vi "get parameters.vi"(8 "error in (no error)":errorcluster, 11 "Request in":variant) -> (0 "error out":errorcluster, 1 "found?":bool, 2 "params":variant, 3 "Request out":variant)   [LabVIEW 2017, in "JSONRPC Server.lvclass"]
uses:
  JSONRPC Server.lvclass
  <vilib>/National Instruments/Variant Data Manipulation/Variant Data Manipulation.lvlib
  <vilib>/Utility/Data Type/NI_Data Type.lvlib
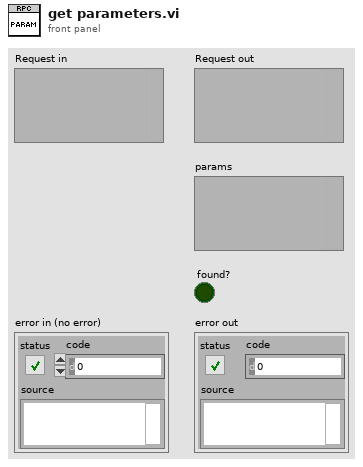
[diagram p1: front panel]
types:
  T1 = typedef "NI_Data Type.lvlib/Data Type.ctl" = enum8{"Invalid Type", "Void", "I8", "I16", "I32", "I64", "U8", "U16", "U32", "U64", "Single Float", "Double Float", "Extended Float", "Single Complex", "Double Complex", "Extended Complex", "Enum U8", "Enum U16", "Enum U32", "Enum U64", "Single Float With Unit", "Double Float With Unit", "Extended Float With Unit", "Single Complex with Unit", "Double Complex with Unit", "Extended Complex with Unit", "Boolean", "String", "Path", "Picture", "Tag", "Array", "Cluster", "Variant", "LV Variant", "Waveform", "Timestamp", "Digital Waveform", "Digital Data", "ExpressData", "Refnum", "External Data", "VI", "Poly VI", "LabVIEW Class Instance", "Fixed Point"}
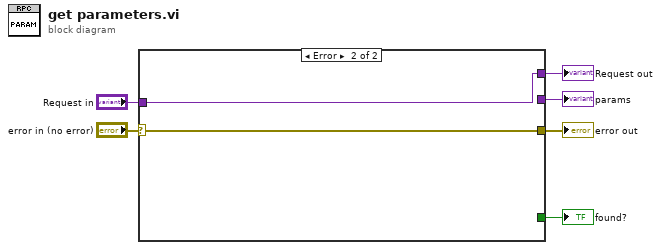
[diagram p0: block diagram]
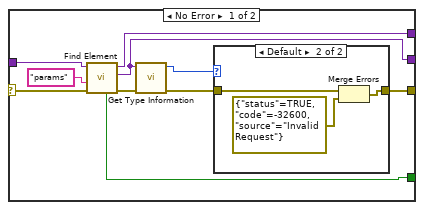
[diagram p2: hidden frame]
diagram:
  n1 = case shown="Error" "error in (no error)" {
    selector: "error in (no error)" -> [w14 w21]
    tunnel: "Request in" -> [w16 w22]
    tunnel: [w12 w22] -> w4
    tunnel: [w11 _] -> w3
    tunnel: [w10 _] -> w2
    tunnel: [w9 w21] -> w1
    frame No Error {
      n2 = call <vilib>:"Find Element.vi"("error in (no error)"=w14, "Name"="params", "Variant (Cluster) in"=w16) -> ("error out"=w15:errorcluster, "element"=w10:variant, "Variant (Cluster) out"=w12:variant, "found?"=w11:bool)  [unwired: 4 in, 1 out]
      n3 = call <vilib>:"Get Type Information.vi"("error in (no error)"=w15, "Variant"=w10) -> ("error out"=w7:errorcluster, "Type"=w8:T1)  [unwired: 5 in, 3 out]
      n4 = case shown="Default" w8 {
        tunnel: [w17 w19] -> w9
        tunnel: w7 -> [w17 w18]
        frame "Void", "Array", "Cluster" {
        }
        frame Default {
          n5 = Merge Errors(w18, errorcluster {"status"=TRUE, "code"=-32600, "source"="Invalid Request"} ("error IO")) -> (w19:errorcluster)
        }
      }
    }
    frame Error {
    }
  }
  "error out" <- w1
  "params" <- w2
  "Request out" <- w4
  "found?" <- w3
